vi "New Redis Pipelining TCP Client.vi"(6 "pipelining enabled?":bool, 8 "error in (no error)":errorcluster, 9 "timeout ms (25000)":i32=25000, 10 "remote port or service name":u16=6379, 11 "address":string) -> (0 "error out":errorcluster, 3 "Redis Pipelining TCP Client out":refnum<class "Redis Pipelining TCP Client.lvclass">)   [LabVIEW 2019, in "Redis Client for LabVIEW.lvlib" / "Redis Pipelining TCP Client.lvclass"]
uses:
  Redis Pipelining TCP Client.lvclass
  Redis Pipelining TCP Client.lvclass/Redis Pipelining TCP Client.ctl
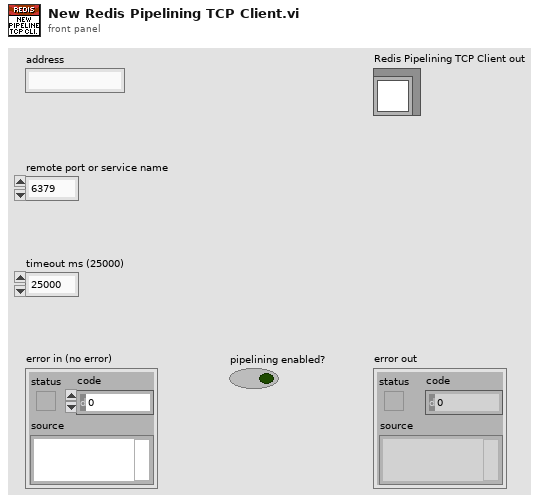
[diagram p1: front panel]
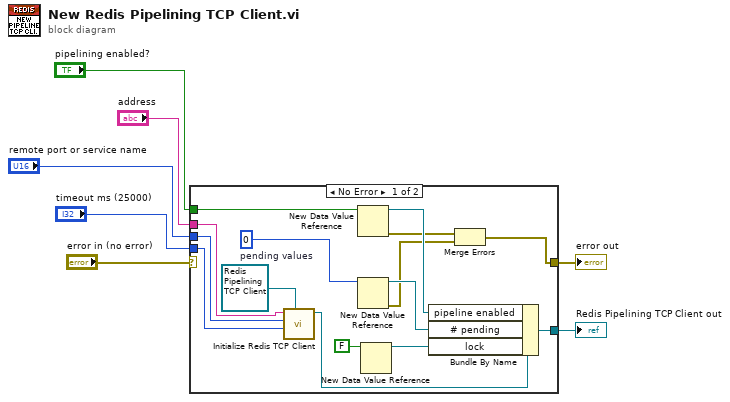
[diagram p0: block diagram]
diagram:
  n1 = case shown="No Error" "error in (no error)" {
    selector: "error in (no error)" -> [_ w23]
    tunnel: [w10 w23] -> w6
    tunnel: [w22 _] -> w1
    tunnel: "address" -> [w21 _]
    tunnel: "remote port or service name" -> [w19 _]
    tunnel: "timeout ms (25000)" -> [w20 _]
    tunnel: "pipelining enabled?" -> [w14 _]
    frame No Error {
      w16 = 0  # pending values
      n2 = call-dynamic "Initialize Redis TCP Client.vi"("Redis TCP Client in"=refnum<class "Redis Pipelining TCP Client.lvclass"> refnum ("Redis Pipelining TCP Client in"), "timeout ms (25000)"=w20, "remote port or service name"=w19, "address"=w21) -> ("Redis TCP Client out"=w18:refnum<class "Redis Pipelining TCP Client.lvclass">)  [unwired: 6 in, 1 out]
      n3 = New Data Value Reference(data value=w14) -> (data value reference=w13:refnum<data-value>, error out=w12:errorcluster)  [unwired: 1 in]
      n4 = New Data Value Reference(data value=w16) -> (data value reference=w15:refnum<data-value>, error out=w11:errorcluster)  [unwired: 1 in]
      n5 = New Data Value Reference(data value=FALSE) -> (data value reference=w9:refnum<data-value>)  [unwired: 1 in, 1 out]
      n6 = Bundle By Name(cluster=w18, "pipeline enabled"=w13, "# pending"=w15, "lock"=w9) -> (w22:refnum<class "Redis Pipelining TCP Client.lvclass">)
      n7 = Merge Errors(w12, w11) -> (w10:errorcluster)
    }
    frame Error {
    }
  }
  "error out" <- w6
  "Redis Pipelining TCP Client out" <- w1
